vi "PID DW.vi"(4 "Init?":bool, 6 "Output Limits":cluster{"Hi":dbl, "Low":dbl}, 7 "Auto/Manual":bool, 8 "dT(in)":dbl, 9 "PID Coefficients":cluster{"P":dbl, "I":dbl, "D":dbl}, 10 "Process Variable":dbl, 11 "Setpoint":dbl) -> (0 "dT":dbl, 2 "Output":dbl)   [LabVIEW 2016]
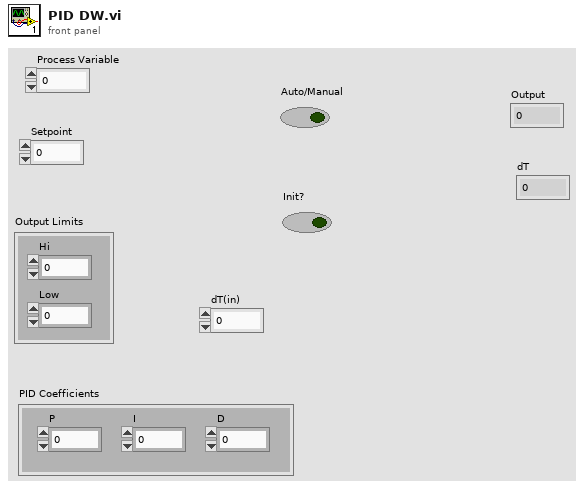
[diagram p1: front panel]
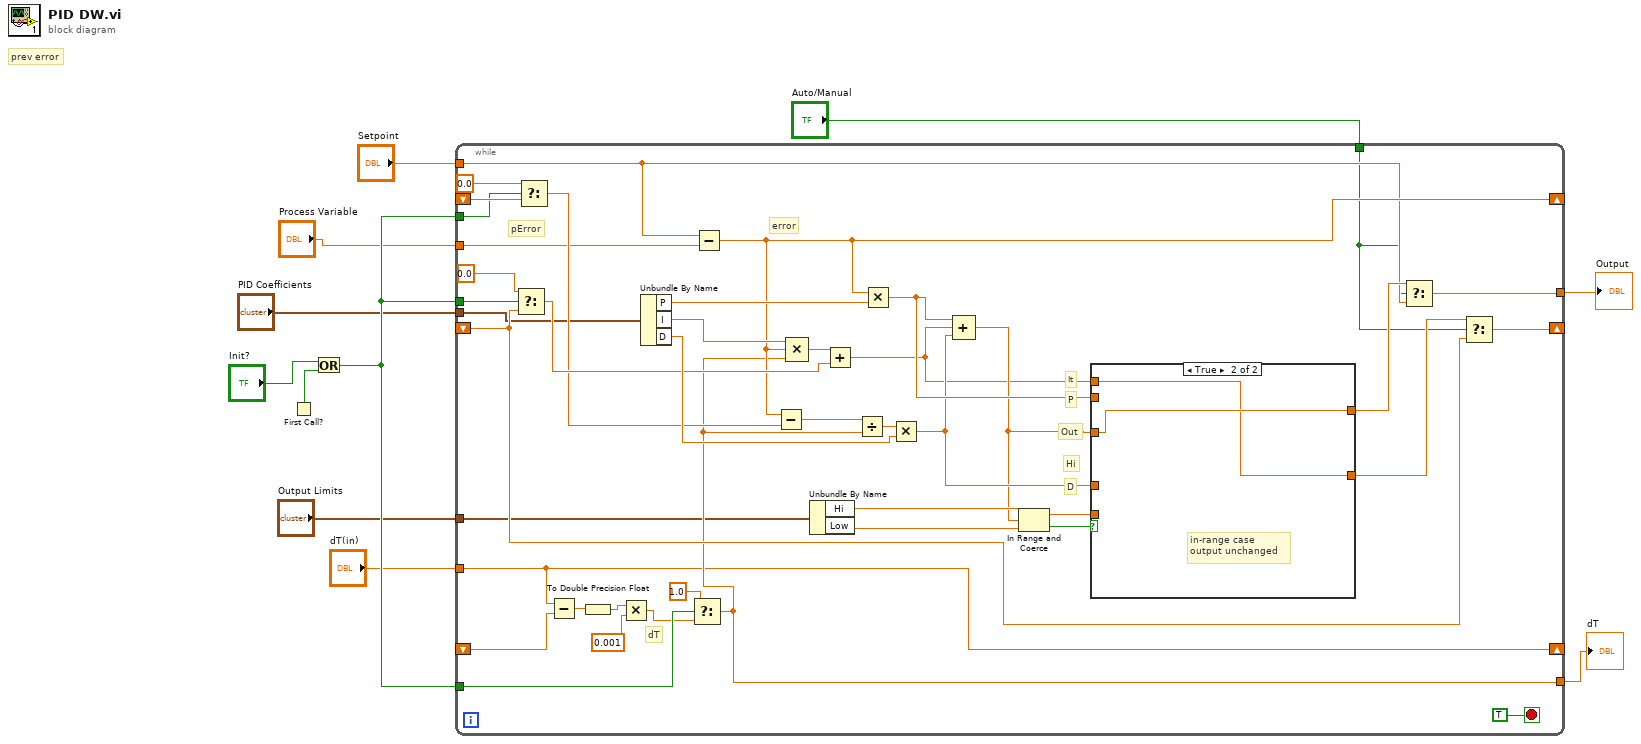
[diagram p0: block diagram]
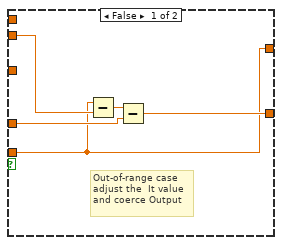
[diagram p2: hidden frame]
diagram:
  # "prev error"
  n1 = First Call?() -> (First Call?: T/F=w10:bool)
  n2 = Or(x="Init?", y=w10) -> (x .or. y?=w8:bool)
  n3 = while {
    shift-right: [w25] -> _
    shift-left: _ -> [w38]
    shift-right: [w28] -> _
    shift-left: _ -> [w26]
    shift-right: [w12] -> _
    shift-left: _ -> [w31]
    tunnel: w8 -> [w36]
    tunnel: w8 -> [w33]
    tunnel: w8 -> [w32]
    tunnel: [w21] -> w11
    tunnel: "Setpoint" -> [w18]
    tunnel: "Process Variable" -> [w17]
    tunnel: "PID Coefficients" -> [w16]
    tunnel: [w15] -> w4
    tunnel: "Auto/Manual" -> [w14]
    tunnel: "Output Limits" -> [w13]
    tunnel: "dT(in)" -> [w12]
    stop <- TRUE stop-if-true
    # "Out"
    # "Hi"
    # "D"
    # "P"
    # "It"
    # "pError"
    # "dT"
    # "error"
    n4 = Select(t=0.0, s=w33, f=w26) -> (s? t:f=w35:dbl)
    n5 = Select(t=0.0, s=w36, f=w38) -> (s? t:f=w24:dbl)
    n6 = Subtract(x=w12, y=w31) -> (x-y=w20:dbl)
    n7 = To Double Precision Float(number=w20) -> (double precision float=w19:dbl)
    n8 = Multiply(x=w19, y=0.001) -> (x*y=w22:dbl)
    n9 = Unbundle By Name(w16) -> ("P"=w53:dbl, "I"=w52:dbl, "D"=w48:dbl)
    n10 = Select(t=sgl 1.0, s=w32, f=w22) -> (s? t:f=w21:dbl)
    n11 = Subtract(x=w18, y=w17) -> (x-y=w25:dbl)
    n12 = Subtract(x=w25, y=w24) -> (x-y=w50:dbl)
    n13 = Compound Arithmetic op=MULTIPLY(w52, w25, w21) -> (w51:dbl)
    n14 = Unbundle By Name(w13) -> ("Hi"=w44:dbl, "Low"=w42:dbl)
    n15 = Add(x=w51, y=w35) -> (x+y=w27:dbl)
    n16 = Divide(x=w50, y=w21) -> (x/y=w49:dbl)
    n17 = Multiply(x=w25, y=w53) -> (x*y=w46:dbl)
    n18 = Multiply(x=w49, y=w48) -> (x*y=w45:dbl)
    n19 = Compound Arithmetic op=ADD(w46, w27, w45) -> (w41:dbl)
    n20 = In Range and Coerce(upper limit=w44, x=w41, lower limit=w42) -> (coerced(x)=w40:dbl, In Range?=w43:bool)
    n21 = case shown="True" w43 {
      tunnel: w46 -> [w58 _]
      tunnel: w45 -> [w56 _]
      tunnel: w27 -> [_ w59]
      tunnel: [w55 w59] -> w29
      tunnel: [w54 w60] -> w39
      tunnel: w41 -> [_ w60]
      tunnel: w40 -> [w54 _]
      frame False {
        # "Out-of-range case\nadjust the  It value \nand coerce Output"
        n22 = Subtract(x=w54, y=w58) -> (x-y=w57:dbl)
        n23 = Subtract(x=w57, y=w56) -> (x-y=w55:dbl)
      }
      frame True {
        # "in-range case\noutput unchanged"
      }
    }
    n24 = Select(t=w39, s=w14, f=w18) -> (s? t:f=w15:dbl)
    n25 = Select(t=w29, s=w14, f=w26) -> (s? t:f=w28:dbl)
  }
  "dT" <- w11
  "Output" <- w4
